vi "Stimulus trig-Funct acq pulse width abs lim.vi"(11 "Funct acq. stimulus trigger pulse width (ms)":dbl) -> (3 "Funct acq. stimulus trigger pulse width (ms)":dbl)   [LabVIEW 2020]
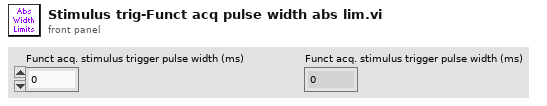
[diagram p1: front panel]
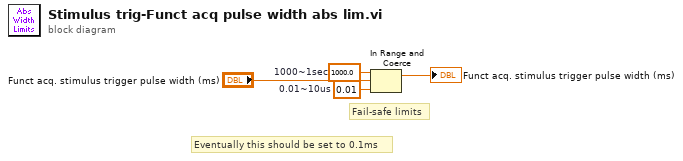
[diagram p0: block diagram]
diagram:
  w1 = 1000.0  # 1000~1sec
  w2 = 0.01  # 0.01~10us
  # "Eventually this should be set to 0.1ms"
  # "Fail-safe limits"
  n1 = In Range and Coerce(upper limit=w1, x="Funct acq. stimulus trigger pulse width (ms)", lower limit=w2) -> (coerced(x)=→"Funct acq. stimulus trigger pulse width (ms)":dbl)  [unwired: 1 out]
